vi "Shutdown.vi"(8 "error in (no error)":errorcluster, 11 "MB in":refnum<class "Modbus Master CR.lvclass">) -> (0 "error out":errorcluster)   [LabVIEW 2021, in "Modbus Master CR.lvclass"]
doc: "Closes and destroys a Modbus master instance."
uses:
  Modbus Master CR.lvclass
  Modbus Master CR.lvclass/Modbus Master CR.ctl
  Network Master/Network Master.lvclass
  Data Model/Device Data Model.lvclass
  MB Param/MB Param/MB Param.lvclass
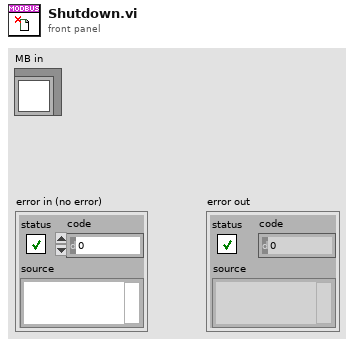
[diagram p1: front panel]
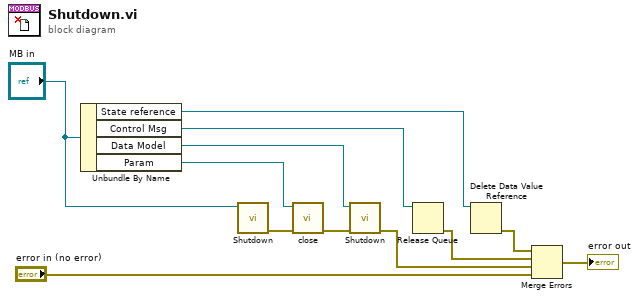
[diagram p0: block diagram]
diagram:
  n1 = Unbundle By Name("MB in") -> ("State reference"=w12:refnum<data-value>, "Control Msg"=w9:refnum<queue>, "Data Model"=w3:refnum<class "Device Data Model.lvclass">, "Param"=w6:refnum<class "MB Param.lvclass">)
  n2 = call-parent "Shutdown.vi"("Network Master in"="MB in") -> ("error out"=w2:errorcluster)  [unwired: 10 in]
  n3 = call-dynamic "close.vi"("error in"=w2, "MBParam in"=w6) -> ("error out"=w5:errorcluster)  [unwired: 9 in]
  n4 = call-dynamic "Shutdown.vi"("error in"=w5, "device data model in"=w3) -> ("error out"=w4:errorcluster)  [unwired: 9 in]
  n5 = Release Queue(queue=w9) -> (error out=w7:errorcluster)  [unwired: 2 in, 2 out]
  n6 = Delete Data Value Reference(data value reference=w12) -> (error out=w10:errorcluster)  [unwired: 1 in, 1 out]
  n7 = Merge Errors(w10, w7, w4, "error in (no error)") -> (→"error out":errorcluster)
